vi "Read Signal Data Start.vi"(8 "error in":errorcluster, 10 "Device":string, 11 "SLL in":refnum<class "SLL.lvclass">) -> (0 "error out":errorcluster, 3 "SLL out":refnum<class "SLL.lvclass">)   [LabVIEW 2023, in "SLL.lvlib" / "SLL.lvclass"]
uses:
  SLL.lvclass
  SLL.lvclass/SLL.ctl
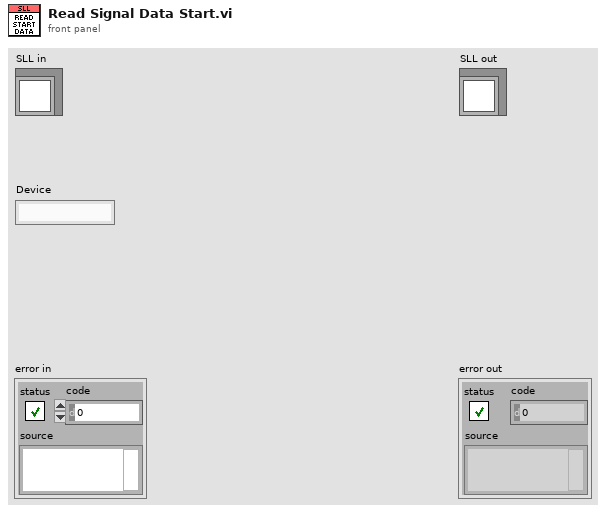
[diagram p1: front panel]
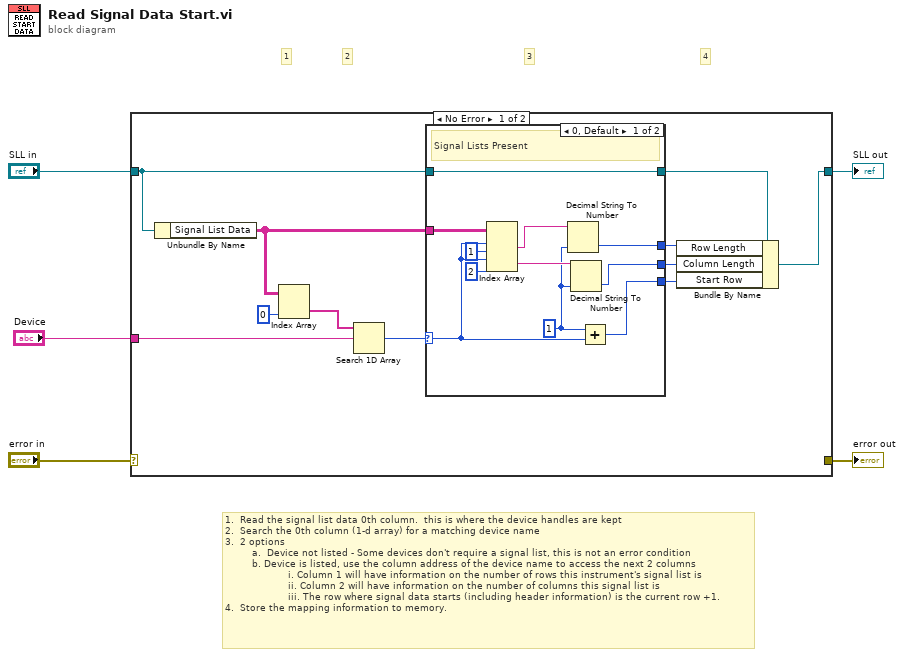
[diagram p0: block diagram]
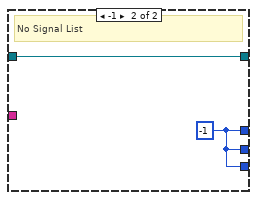
[diagram p2: hidden frame]
diagram:
  # "1.  Read the signal list data 0th column.  this is where the device handles are kept\n2.  Search the 0th column (1-d array) for a matching device name\n3.  2 options\n         a.  Device not listed - Some devices don't require a signal list, this is not an error condition\n         b. Device is listed, use the column address of the device name to access the next 2 columns\n                     i. Column 1 will have information on the number of rows this instrument's signal list is\n                     ii. Column 2 will have information on the number of columns this signal list is\n                     iii. The row where signal data starts (including header information) is the current row +1.\n4.  Store the mapping information to memory."
  # "4"
  # "3"
  # "2"
  # "1"
  n1 = case shown="No Error" "error in" {
    selector: "error in" -> [_ w31]
    tunnel: [_ w31] -> w4
    tunnel: [w7 w30] -> w2
    tunnel: "SLL in" -> [w11 w30]
    tunnel: "Device" -> [w14 _]
    frame No Error {
      n2 = Unbundle By Name(w11) -> ("Signal List Data"=w12:string[][])
      n3 = Index Array(array=w12, index (col)=0 ("disabled index (col)")) -> (element=w15:string[])  [unwired: 1 in]
      n4 = Search 1D Array(1D array=w15, element=w14) -> (index of element=w13:i32)  [unwired: 1 in]
      n5 = case shown="0, Default" w13 {
        selector: w13 -> [w19 _]
        tunnel: w12 -> [w27 _]
        tunnel: w11 -> [w21 w29]
        tunnel: [w21 w29] -> w8
        tunnel: [w17 w28] -> w10
        tunnel: [w22 w28] -> w9
        tunnel: [w18 w28] -> w6
        frame 0, Default {
          w20 = 1 ("disabled index (col)")
          # "Signal Lists Present"
          n6 = Index Array(array=w27, index (row) #1=w19, index (col) #1=1 ("disabled index (col)"), index (row) #2=w19, index (col) #2=2 ("disabled index (col)")) -> (element #1=w23:string, element #2=w24:string)
          n7 = Decimal String To Number(string=w23, default (0L)=w20) -> (number=w17:i32)  [unwired: 1 in, 1 out]
          n8 = Decimal String To Number(string=w24, default (0L)=w20) -> (number=w22:i32)  [unwired: 1 in, 1 out]
          n9 = Add(x=w20, y=w19) -> (x+y=w18:i32)
        }
        frame -1 {
          w28 = -1
          # "No Signal List"
        }
      }
      n10 = Bundle By Name(cluster=w8, "Row Length"=w10, "Column Length"=w9, "Start Row"=w6) -> (w7:refnum<class "SLL.lvclass">)
    }
    frame Error {
    }
  }
  "error out" <- w4
  "SLL out" <- w2
